vi "Calculate Center.vi"(8 "Type of Assembly Tray":i32, 9 "Syringe Coordinates":dbl[](array[numeric]), 10 "Relative Coordinates":dbl[][](array[numeric]), 11 "Fiducial Measurements":dbl[][](array[numeric])) -> (3 "XYZTheta Centers":dbl[][](array[numeric]) format="%#.9g")   [LabVIEW 2020, in "Assembly Tray.lvclass"]
uses:
  Assembly Tray.lvclass
  <vilib>/Analysis/NI_AALPro.lvlib
  <vilib>/Analysis/coordinate.llb/2D Cartesian Coordinate Rotation (Scalar).vi
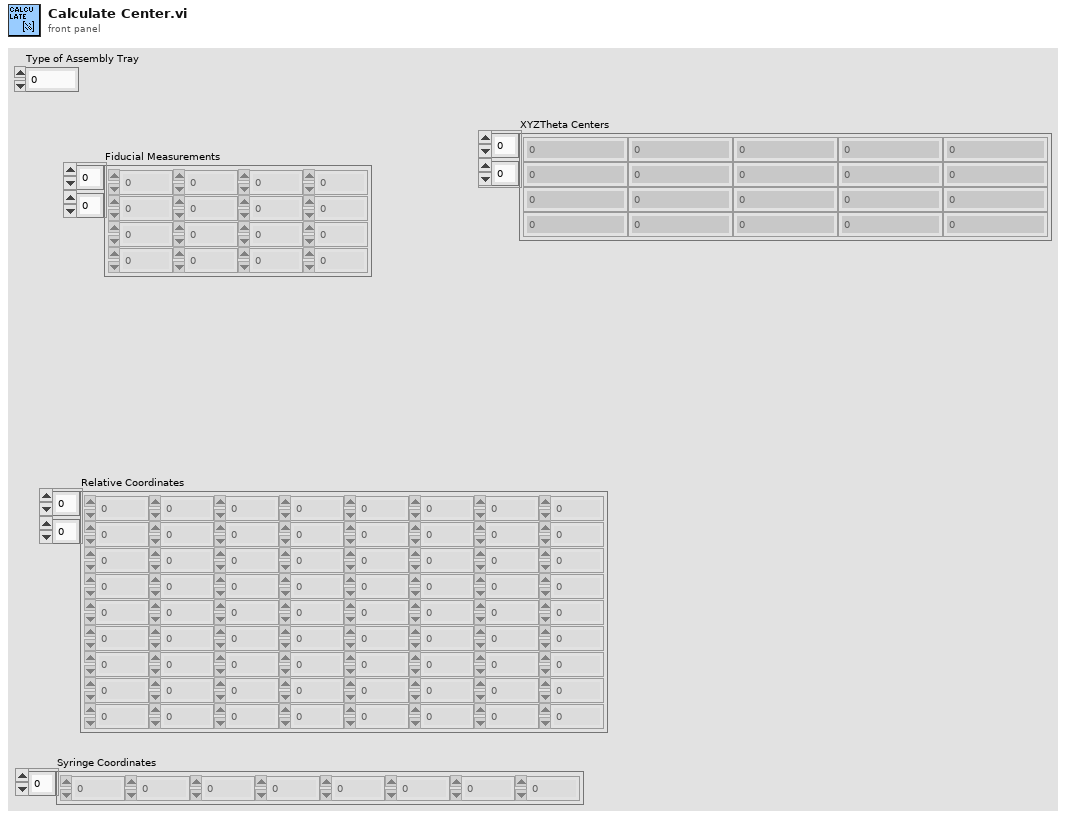
[diagram p1: front panel]
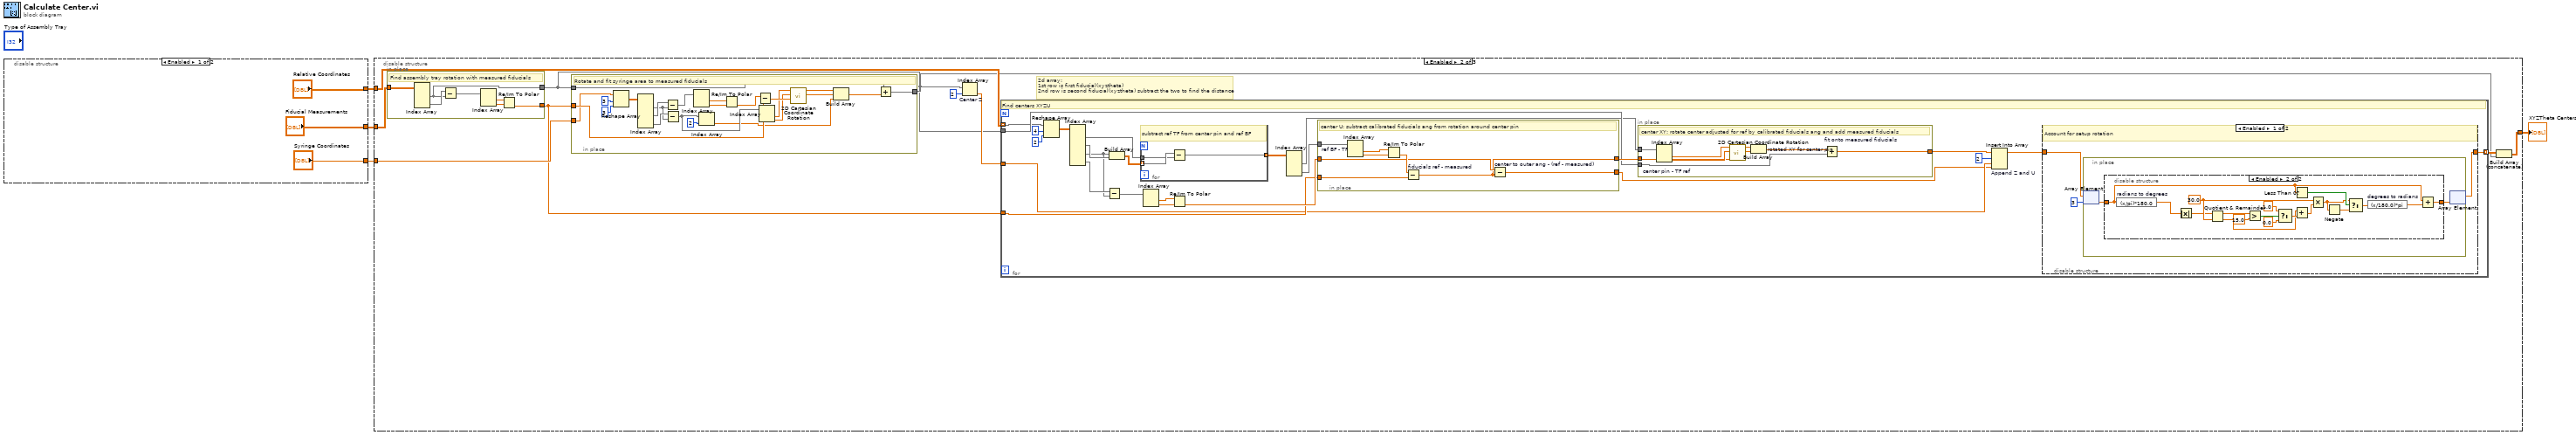
[diagram p0: block diagram]
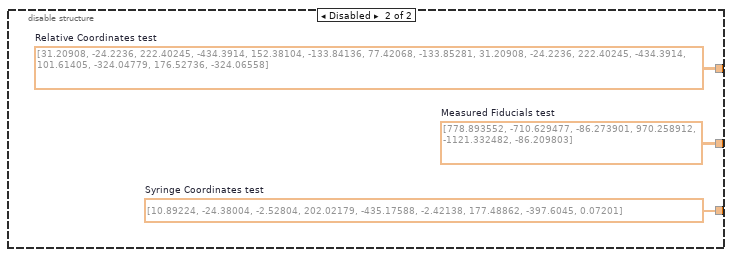
[diagram p2: hidden frame]
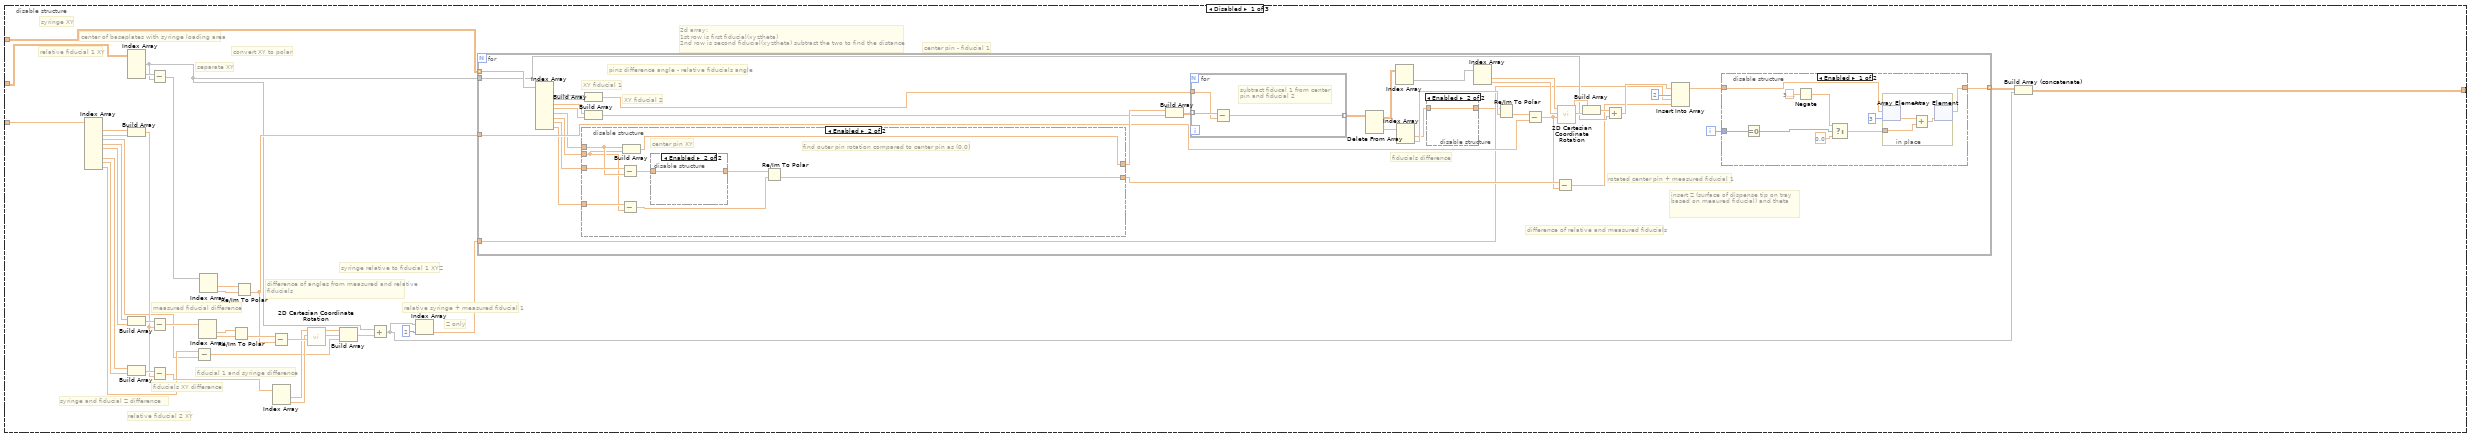
[diagram p3: hidden frame]
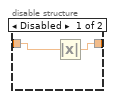
[diagram p4: hidden frame]
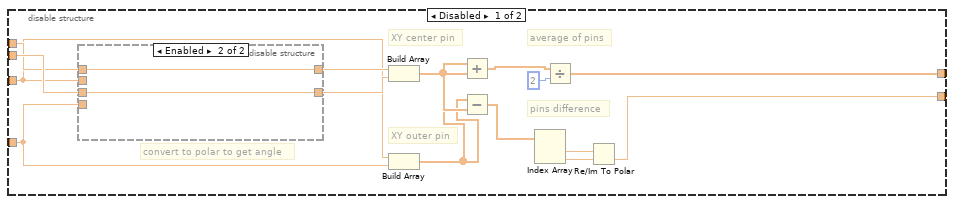
[diagram p5: hidden frame]
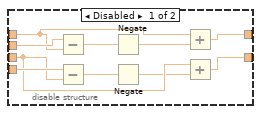
[diagram p6: hidden frame]
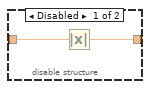
[diagram p7: hidden frame]
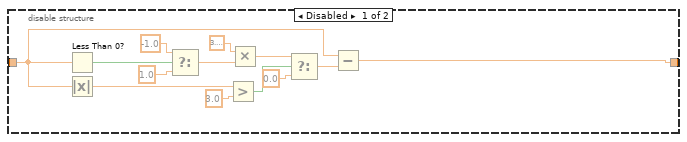
[diagram p9: hidden frame]
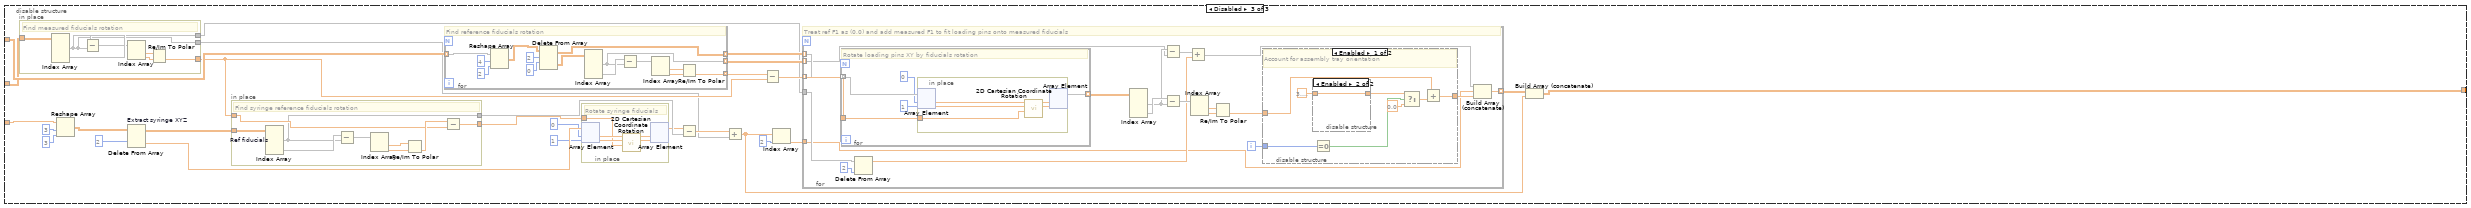
[diagram p11: hidden frame]
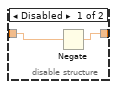
[diagram p12: hidden frame]
diagram:
  n1 = disable-structure shown="Enabled" {
    disable-tunnel: ["Syringe Coordinates" w8] -> w3
    disable-tunnel: ["Fiducial Measurements" w9] -> w2
    disable-tunnel: ["Relative Coordinates" w10] -> w1
    frame Enabled {
    }
    frame Disabled {
      w8 = dbl[] [10.89224, -24.38004, -2.52804, 202.02179, -435.17588, -2.42138, 177.48862, -397.6045, 0.07201]  # Syringe Coordinates test
      w9 = dbl[][] [[778.893552, -710.629477, -86.273901], [970.258912, -1121.332482, -86.209803]]  # Measured Fiducials test
      w10 = dbl[][] [[31.20908, -24.2236, 222.40245, -434.3914, 152.38104, -133.84136, 77.42068, -133.85281], [31.20908, -24.2236, 222.40245, -434.3914, 101.61405, -324.04779, 176.52736, -324.06558]]  # Relative Coordinates test
    }
  }
  n2 = disable-structure shown="Enabled" {
    disable-tunnel: w1 -> [w47 w152 w291]
    disable-tunnel: w2 -> [w44 w151 w290]
    disable-tunnel: w3 -> [w43 w150 w284]
    disable-tunnel: [w19 w147 w269] -> w4
    frame Disabled {
      # "center of baseplates with syringe loading area"
      # "relative fiducial 2 XY"
      # "relative fiducial 1 XY"
      # "syringe XY"
      # "center pin - fiducial 1"
      # "Z only"
      # "relative syringe + measured fiducial 1"
      # "syringe relative to fiducial 1 XYZ"
      # "difference of angles from measured and relative fiducials"
      # "separate XY"
      # "convert XY to polar"
      # "measured fiducial difference"
      # "fiducial 1 and syringe difference"
      # "syringe and fiducial Z difference"
      # "fiducials XY difference"
      # "2d array:\n1st row is first fiducial(xyztheta)\n2nd row is second fiducial(xyztheta) subtract the two to find the distance"
      n3 = Index Array(array=w43) -> (element #1=w42:dbl, element #2=w41:dbl, element #3=w23:dbl, element #4=w39:dbl, element #5=w38:dbl, element #7=w26:dbl, element #8=w25:dbl, element #9=w24:dbl)  [unwired: 9 in, 1 out]
      n4 = Index Array(array=w44) -> (element #1=w11:dbl[], element #2=w13:dbl[])  [unwired: 4 in]
      n5 = Build Array(w42, w41) -> (w30:dbl[])
      n6 = Build Array(w39, w38) -> (w40:dbl[])
      n7 = Build Array(w26, w25) -> (w31:dbl[])
      n8 = Subtract(x=w13, y=w11) -> (x-y=w18:dbl[])
      n9 = Subtract(x=w40, y=w30) -> (x-y=w37:dbl[])
      n10 = Subtract(x=w31, y=w30) -> (x-y=w29:dbl[])
      n11 = Subtract(x=w24, y=w23) -> (x-y=w15:dbl)
      n12 = Index Array(array=w37) -> (element #1=w36:dbl, element #2=w35:dbl)  [unwired: 2 in]
      n13 = Index Array(array=w18) -> (element #1=w45:dbl, element #2=w46:dbl)  [unwired: 2 in]
      n14 = Re/Im To Polar(2:w35, 3:w36) -> (0:w34:dbl)  [unwired: 1 out]
      n15 = Re/Im To Polar(2:w46, 3:w45) -> (0:w33:dbl)  [unwired: 1 out]
      n16 = Subtract(x=w34, y=w33) -> (x-y=w32:dbl)
      n17 = Index Array(array=w29) -> (element #1=w28:dbl, element #2=w27:dbl)  [unwired: 2 in]
      n18 = call-poly <vilib>:"2D Cartesian Coordinate Rotation.vi"("theta"=w32, "y"=w27, "x"=w28) -> ("y out"=w21:dbl, "x out"=w22:dbl)  [unwired: 6 in, 1 out]
      n19 = Build Array(w22, w21, w15) -> (w12:dbl[])
      n20 = Add(x=w11, y=w12) -> (x+y=w14:dbl[])
      n21 = Index Array(array=w14, index=2) -> (element=w16:dbl)
      n22 = for {
        tunnel: w47 -> [w64] mode=indexing
        tunnel: [w55] -> w20 mode=indexing
        tunnel: w11 -> [w63]
        tunnel: w33 -> [w62]
        tunnel: w16 -> [w61]
        i -> [w54]
        # "insert Z (surface of dispense tip on tray based on meaured fiducial) and theta"
        # "pins difference angle - relative fiducials angle"
        # "rotated center pin + measured fiducial 1"
        # "difference of relative and measured fiducials"
        # "fiducials difference"
        # "XY fiducial 2"
        # "XY fiducial 1"
        n23 = Index Array(array=w64) -> (element #1=w84:dbl, element #2=w83:dbl, element #3=w53:dbl, element #4=w52:dbl, element #5=w59:dbl, element #6=w60:dbl, element #7=w58:dbl, element #8=w57:dbl)  [unwired: 8 in]
        n24 = disable-structure shown="Enabled" {
          disable-tunnel: [w100 w115] -> w68
          disable-tunnel: [w94 w119] -> w66
          disable-tunnel: w60 -> [w91 w116]
          disable-tunnel: w59 -> [w90 w117]
          disable-tunnel: w58 -> [w89 w120]
          disable-tunnel: w57 -> [w88 w118]
          frame Disabled {
            # "convert to polar to get angle"
            # "pins difference"
            # "average of pins"
            # "XY outer pin"
            # "XY center pin"
            n25 = disable-structure shown="Enabled" {
              disable-tunnel: w88 -> [w112 _]
              disable-tunnel: w89 -> [w111 _]
              disable-tunnel: w91 -> [w108 w114]
              disable-tunnel: w90 -> [w105 w113]
              disable-tunnel: [w104 w114] -> w92
              disable-tunnel: [w103 w113] -> w93
              frame Disabled {
                n26 = Subtract(x=w111, y=w105) -> (x-y=w109:dbl)
                n27 = Subtract(x=w112, y=w108) -> (x-y=w110:dbl)
                n28 = Negate(x=w109) -> (-x=w106:dbl)
                n29 = Negate(x=w110) -> (-x=w107:dbl)
                n30 = Add(x=w105, y=w106) -> (x+y=w103:dbl)
                n31 = Add(x=w108, y=w107) -> (x+y=w104:dbl)
              }
              frame Enabled {
              }
            }
            n32 = Build Array(w93, w92) -> (w99:dbl[])
            n33 = Build Array(w89, w88) -> (w98:dbl[])
            n34 = Add(x=w98, y=w99) -> (x+y=w101:dbl[])
            n35 = Subtract(x=w98, y=w99) -> (x-y=w97:dbl[])
            n36 = Index Array(array=w97) -> (element #1=w96:dbl, element #2=w95:dbl)  [unwired: 2 in]
            n37 = Divide(x=w101, y=2) -> (x/y=w100:dbl[])
            n38 = Re/Im To Polar(2:w95, 3:w96) -> (0:w94:dbl)  [unwired: 1 out]
          }
          frame Enabled {
            # "find outer pin rotation compared to center pin as (0,0)"
            # "center pin XY"
            n39 = Subtract(x=w120, y=w117) -> (x-y=w122:dbl)
            n40 = Subtract(x=w118, y=w116) -> (x-y=w123:dbl)
            n41 = Build Array(w117, w116) -> (w115:dbl[])
            n42 = disable-structure shown="Enabled" {
              disable-tunnel: w122 -> [w125 w126]
              disable-tunnel: [w124 w126] -> w121
              frame Disabled {
                n43 = Absolute Value(x=w125) -> (abs(x)=w124:dbl)
              }
              frame Enabled {
              }
            }
            n44 = Re/Im To Polar(2:w123, 3:w121) -> (0:w119:dbl)  [unwired: 1 out]
          }
        }
        n45 = Build Array(w84, w83) -> (w81:dbl[])
        n46 = Build Array(w53, w52) -> (w51:dbl[])
        n47 = Build Array(w68, w51) -> (w82:dbl[][])
        n48 = for {
          tunnel: w82 -> [w142] mode=indexing
          tunnel: w81 -> [w141]
          tunnel: [w140] -> w80 mode=indexing
          # "subtract fiducal 1 from center pin and fiducial 2"
          n49 = Subtract(x=w142, y=w141) -> (x-y=w140:dbl[])
        }
        n50 = Delete From Array(array=w80) -> (deleted portion=w79:dbl[], array with subset deleted=w77:dbl[][])  [unwired: 3 in]
        n51 = Index Array(array=w77) -> (element=w76:dbl[])  [unwired: 2 in]
        n52 = Index Array(array=w79) -> (element #1=w50:dbl, element #2=w78:dbl)  [unwired: 2 in]
        n53 = disable-structure shown="Enabled" {
          disable-tunnel: w50 -> [w86 w87]
          disable-tunnel: [w85 w87] -> w49
          frame Disabled {
            n54 = Absolute Value(x=w86) -> (abs(x)=w85:dbl)
          }
          frame Enabled {
          }
        }
        n55 = Index Array(array=w76) -> (element #1=w75:dbl, element #2=w74:dbl)  [unwired: 2 in]
        n56 = Re/Im To Polar(2:w78, 3:w49) -> (0:w67:dbl)  [unwired: 1 out]
        n57 = Subtract(x=w67, y=w62) -> (x-y=w65:dbl)
        n58 = Subtract(x=w66, y=w65) -> (x-y=w48:dbl)
        n59 = call-poly <vilib>:"2D Cartesian Coordinate Rotation.vi"("theta"=w65, "y"=w74, "x"=w75) -> ("y out"=w71:dbl, "x out"=w72:dbl)  [unwired: 6 in, 1 out]
        n60 = Build Array(w72, w71) -> (w73:dbl[])
        n61 = Add(x=w73, y=w63) -> (x+y=w70:dbl[])
        n62 = Insert Into Array(array=w70, index=2, new element #1=w61, new element #2=w48) -> (w56:dbl[])
        n63 = disable-structure shown="Enabled" {
          disable-tunnel: w56 -> [w135 w139]
          disable-tunnel: [w134 w139] -> w55
          disable-tunnel: w54 -> [w132 _]
          frame Enabled {
            n64 = Equal To 0?(x=w132) -> (x = 0?=w130:bool)
            n65 = Negate(x=3.141592653589793) -> (-x=w127:dbl)
            n66 = Select(t=w127, s=w130, f=0.0) -> (s? t:f=w129:dbl)
            n67 = in-place {
              in-place-border: w129 -> [w136]
              n68 = in-place-array #1(w135, 3) -> (w138:dbl)
              n69 = Add(x=w138, y=w136) -> (x+y=w137:dbl)
              n70 = in-place-array #1(w137) -> (w134:dbl[])  [unwired: 1 out]
            }
          }
          frame Disabled {
          }
        }
      }
      n71 = Build Array (concatenate)(w20, w14) -> (w19:dbl[][])
    }
    frame Enabled {
      # "2d array:\n1st row is first fiducial(xyztheta)\n2nd row is second fiducial(xyztheta) subtract the two to find the distance"
      n72 = in-place {
        in-place-border: w151 -> [w239]
        in-place-border: [w238] -> w149
        in-place-border: [w235] -> w143
        # "Find assembly tray rotation with measured fiducials"
        n73 = Index Array(array=w239) -> (element #1=w235:dbl[], element #2=w236:dbl[])  [unwired: 4 in]
        n74 = Subtract(x=w236, y=w235) -> (x-y=w237:dbl[])
        n75 = Index Array(array=w237) -> (element #1=w240:dbl, element #2=w241:dbl)  [unwired: 2 in]
        n76 = Re/Im To Polar(2:w241, 3:w240) -> (0:w238:dbl)  [unwired: 1 out]
      }
      n77 = in-place {
        in-place-border: w150 -> [w252]
        in-place-border: w149 -> [w261]
        in-place-border: [w255] -> w144
        in-place-border: w143 -> [w253]
        # "Rotate and fit syringe area to measured fiducials"
        n78 = Reshape Array(w252, 3 ("dimension size"), 3 ("dimension size")) -> (w249:dbl[][])
        n79 = Index Array(array=w249) -> (element #1=w246:dbl[], element #2=w248:dbl[], element #3=w247:dbl[])  [unwired: 6 in]
        n80 = Subtract(x=w248, y=w246) -> (x-y=w245:dbl[])
        n81 = Subtract(x=w247, y=w246) -> (x-y=w244:dbl[])
        n82 = Index Array(array=w245) -> (element #1=w264:dbl, element #2=w263:dbl)  [unwired: 2 in]
        n83 = Index Array(array=w244, index=2) -> (element=w242:dbl)
        n84 = Re/Im To Polar(2:w263, 3:w264) -> (0:w262:dbl)  [unwired: 1 out]
        n85 = Subtract(x=w262, y=w261) -> (x-y=w260:dbl)
        n86 = Index Array(array=w244) -> (element #1=w259:dbl, element #2=w258:dbl)  [unwired: 2 in]
        n87 = call-poly <vilib>:"2D Cartesian Coordinate Rotation.vi"("theta"=w260, "y"=w258, "x"=w259) -> ("y out"=w256:dbl, "x out"=w257:dbl)  [unwired: 6 in, 1 out]
        n88 = Build Array(w257, w256, w242) -> (w254:dbl[])
        n89 = Add(x=w253, y=w254) -> (x+y=w255:dbl[])
      }
      n90 = Index Array "Center Z"(array=w144, index=2) -> (element=w145:dbl)
      n91 = for {
        tunnel: w152 -> [w166] mode=indexing
        tunnel: [w168] -> w148 mode=indexing
        tunnel: w143 -> [w172]
        tunnel: w149 -> [w171]
        tunnel: w145 -> [w170]
        # "Find centers XYZU"
        n92 = Reshape Array(w166, 4 ("dimension size"), 2 ("dimension size")) -> (w163:dbl[][])
        n93 = Index Array(array=w163) -> (element #1=w158:dbl[], element #2=w157:dbl[], element #3=w156:dbl[], element #4=w162:dbl[])  [unwired: 8 in]
        n94 = Subtract(x=w162, y=w156) -> (x-y=w161:dbl[])
        n95 = Build Array(w156, w157) -> (w177:dbl[][])
        n96 = for {
          tunnel: w177 -> [w234] mode=indexing
          tunnel: w158 -> [w233]
          tunnel: [w232] -> w155 mode=indexing
          # "subtract ref TF from center pin and ref BF"
          n97 = Subtract(x=w234, y=w233) -> (x-y=w232:dbl[])
        }
        n98 = Index Array(array=w161) -> (element #1=w160:dbl, element #2=w159:dbl)  [unwired: 2 in]
        n99 = Re/Im To Polar(2:w159, 3:w160) -> (0:w174:dbl)  [unwired: 1 out]
        n100 = Index Array(array=w155) -> (element #1=w154:dbl[], element #2=w153:dbl[])  [unwired: 4 in]
        n101 = in-place {
          in-place-border: w174 -> [w183]
          in-place-border: [w182] -> w173
          in-place-border: w171 -> [w181]
          in-place-border: [w179] -> w167
          in-place-border: w153 -> [w178]
          # "center U: subtract calibrated fiducials ang from rotation around center pin"
          n102 = Index Array "ref BF - TF"(array=w178) -> (element #1=w180:dbl, element #2=w185:dbl)  [unwired: 2 in]
          n103 = Re/Im To Polar(2:w185, 3:w180) -> (0:w184:dbl)  [unwired: 1 out]
          n104 = Subtract "fiducials ref - measured"(x=w184, y=w181) -> (x-y=w182:dbl)
          n105 = Subtract "center to outer ang - (ref - measured)"(x=w183, y=w182) -> (x-y=w179:dbl)
        }
        n106 = in-place {
          in-place-border: [w189] -> w176
          in-place-border: w173 -> [w188]
          in-place-border: w172 -> [w187]
          in-place-border: w154 -> [w186]
          # "center XY: rotate center adjusted for ref by calibrated fiducials ang and add measured fiducials"
          n107 = Index Array "center pin - TF ref"(array=w186) -> (element #1=w194:dbl, element #2=w193:dbl)  [unwired: 2 in]
          n108 = call-poly <vilib>:"2D Cartesian Coordinate Rotation.vi"("theta"=w188, "y"=w193, "x"=w194) -> ("y out"=w190:dbl, "x out"=w191:dbl)  [unwired: 6 in, 1 out]
          n109 = Build Array "rotated XY for center pin"(w191, w190) -> (w192:dbl[])
          n110 = Add "fit onto measured fiducials"(x=w192, y=w187) -> (x+y=w189:dbl[])
        }
        n111 = Insert Into Array "Append Z and U"(array=w176, index=2, new element #1=w170, new element #2=w167) -> (w169:dbl[])
        n112 = disable-structure shown="Enabled" {
          disable-tunnel: w169 -> [w196 w231]
          disable-tunnel: [w195 w231] -> w168
          frame Enabled {
            # "Account for setup rotation"
            n113 = in-place {
              n114 = in-place-array #2(w196, 3) -> (w199:dbl)
              n115 = disable-structure shown="Enabled" {
                disable-tunnel: w199 -> [w206 w216]
                disable-tunnel: [w205 w215] -> w198
                frame Disabled {
                  n116 = Less Than 0?(x=w206) -> (x < 0?=w212:bool)
                  n117 = Absolute Value(x=w206) -> (abs(x)=w209:dbl)
                  n118 = Select(t=-1.0, s=w212, f=1.0) -> (s? t:f=w201:dbl)
                  n119 = Greater?(x=w209, y=3.0) -> (0:w207:bool)
                  n120 = Multiply(x=3.141592653589793, y=w201) -> (x*y=w200:dbl)
                  n121 = Select(t=w200, s=w207, f=0.0) -> (s? t:f=w203:dbl)
                  n122 = Subtract(x=w206, y=w203) -> (x-y=w205:dbl)
                }
                frame Enabled {
                  w223 = 30.0 ("y")
                  n123 = expression code="(x/pi)*180.0" "radians to degrees"(w216) -> (w214:dbl)
                  n124 = Absolute Value(x=w214) -> (abs(x)=w213:dbl)
                  n125 = Quotient & Remainder(x=w213, y=w223) -> (x-y*floor(x/y)=w230:dbl, floor(x/y)=w224:dbl)
                  n126 = Greater?(x=w230, y=15.0) -> (0:w228:bool)
                  n127 = Select(t=1.0, s=w228, f=0.0) -> (s? t:f=w225:dbl)
                  n128 = Less Than 0?(x=w216) -> (x < 0?=w221:bool)
                  n129 = Add(x=w224, y=w225) -> (x+y=w222:dbl)
                  n130 = Multiply(x=w223, y=w222) -> (x*y=w220:dbl)
                  n131 = Negate(x=w220) -> (-x=w219:dbl)
                  n132 = Select(t=w220, s=w221, f=w219) -> (s? t:f=w218:dbl)
                  n133 = expression code="(x/180.0)*pi" "degrees to radians"(w218) -> (w217:dbl)
                  n134 = Add(x=w216, y=w217) -> (x+y=w215:dbl)
                }
              }
              n135 = in-place-array #2(w198) -> (w195:dbl[])  [unwired: 1 out]
            }
          }
          frame Disabled {
          }
        }
      }
      n136 = Build Array (concatenate)(w148, w144) -> (w147:dbl[][])
    }
    frame Disabled {
      n137 = in-place {
        in-place-border: w290 -> [w306]
        in-place-border: [w308] -> w281
        in-place-border: [w307] -> w285
        in-place-border: [w307] -> w271
        # "Find measured fiducials rotation"
        n138 = Index Array(array=w306) -> (element #1=w307:dbl[], element #2=w312:dbl[])  [unwired: 4 in]
        n139 = Subtract(x=w312, y=w307) -> (x-y=w311:dbl[])
        n140 = Index Array(array=w311) -> (element #1=w310:dbl, element #2=w309:dbl)  [unwired: 2 in]
        n141 = Re/Im To Polar(2:w309, 3:w310) -> (0:w308:dbl)  [unwired: 1 out]
      }
      n142 = Reshape Array(w284, 3 ("dimension size"), 3 ("dimension size")) -> (w280:dbl[][])
      n143 = Delete From Array "Extract syringe XYZ"(array=w280, index (row)=2) -> (deleted portion=w277:dbl[], array with subset deleted=w278:dbl[][])  [unwired: 2 in]
      n144 = in-place {
        in-place-border: w281 -> [w300]
        in-place-border: w278 -> [w299]
        in-place-border: [w298] -> w274
        in-place-border: [w297] -> w273
        # "Find syringe reference fiducials rotation"
        n145 = Index Array "Ref fiducials"(array=w299) -> (element #1=w297:dbl[], element #2=w305:dbl[])  [unwired: 4 in]
        n146 = Subtract(x=w305, y=w297) -> (x-y=w304:dbl[])
        n147 = Index Array(array=w304) -> (element #1=w303:dbl, element #2=w302:dbl)  [unwired: 2 in]
        n148 = Re/Im To Polar(2:w302, 3:w303) -> (0:w301:dbl)  [unwired: 1 out]
        n149 = Subtract(x=w301, y=w300) -> (x-y=w298:dbl)
      }
      n150 = for {
        tunnel: w291 -> [w367] mode=indexing
        tunnel: [w360] -> w289 mode=indexing
        tunnel: [w359] -> w286 mode=indexing
        tunnel: [w355] -> w287 mode=indexing
        # "Find reference fiducials rotation"
        n151 = Reshape Array(w367, 4 ("dimension size"), 2 ("dimension size")) -> (w358:dbl[][])
        n152 = Delete From Array(array=w358, length=2, index (row)=0) -> (deleted portion=w354:dbl[][], array with subset deleted=w355:dbl[][])  [unwired: 1 in]
        n153 = Index Array(array=w354) -> (element #1=w359:dbl[], element #2=w364:dbl[])  [unwired: 4 in]
        n154 = Subtract(x=w364, y=w359) -> (x-y=w363:dbl[])
        n155 = Index Array(array=w363) -> (element #1=w362:dbl, element #2=w361:dbl)  [unwired: 2 in]
        n156 = Re/Im To Polar(2:w361, 3:w362) -> (0:w360:dbl)  [unwired: 1 out]
      }
      n157 = in-place {
        in-place-border: w274 -> [w294]
        # "Rotate syringe fiducials"
        n158 = in-place-array #3(w277, 0, 1) -> (w296:dbl, w295:dbl)
        n159 = call-poly <vilib>:"2D Cartesian Coordinate Rotation.vi"("theta"=w294, "y"=w295, "x"=w296) -> ("y out"=w292:dbl, "x out"=w293:dbl)  [unwired: 6 in, 1 out]
        n160 = in-place-array #3(w293, w292) -> (w270:dbl[])  [unwired: 2 out]
      }
      n161 = Subtract(x=w270, y=w273) -> (x-y=w272:dbl[])
      n162 = Add(x=w272, y=w271) -> (x+y=w267:dbl[])
      n163 = Subtract(x=w289, y=w281) -> (x-y=w288:dbl[])
      n164 = Index Array(array=w267, index=2) -> (element=w265:dbl)
      n165 = for {
        tunnel: w288 -> [w331] mode=indexing
        tunnel: w287 -> [w330] mode=indexing
        tunnel: [w324] -> w268 mode=indexing
        tunnel: w286 -> [w317] mode=indexing
        tunnel: w285 -> [w316]
        tunnel: w265 -> [w313]
        i -> [w323]
        # "Treat ref F1 as (0,0) and add measured F1 to fit loading pins onto measured fiducials"
        n166 = for {
          tunnel: w331 -> [w348]
          tunnel: w330 -> [w347] mode=indexing
          tunnel: [w344] -> w329 mode=indexing
          # "Rotate loading pins XY by fiducials rotation"
          n167 = in-place {
            in-place-border: w348 -> [w353]
            n168 = in-place-array #4(w347, 0, 1) -> (w352:dbl, w351:dbl)
            n169 = call-poly <vilib>:"2D Cartesian Coordinate Rotation.vi"("theta"=w353, "y"=w351, "x"=w352) -> ("y out"=w349:dbl, "x out"=w350:dbl)  [unwired: 6 in, 1 out]
            n170 = in-place-array #4(w350, w349) -> (w344:dbl[])  [unwired: 2 out]
          }
        }
        n171 = Delete From Array(array=w316, index=2) -> (array with subset deleted=w314:dbl[])  [unwired: 1 in, 1 out]
        n172 = Index Array(array=w329) -> (element #1=w318:dbl[], element #2=w328:dbl[])  [unwired: 4 in]
        n173 = Subtract(x=w318, y=w317) -> (x-y=w320:dbl[])
        n174 = Subtract(x=w328, y=w318) -> (x-y=w327:dbl[])
        n175 = Add(x=w320, y=w314) -> (x+y=w319:dbl[])
        n176 = Index Array(array=w327) -> (element #1=w326:dbl, element #2=w325:dbl)  [unwired: 2 in]
        n177 = Re/Im To Polar(2:w325, 3:w326) -> (0:w322:dbl)  [unwired: 1 out]
        n178 = disable-structure shown="Enabled" {
          disable-tunnel: w323 -> [w337 _]
          disable-tunnel: w322 -> [w336 w343]
          disable-tunnel: [w334 w343] -> w321
          frame Enabled {
            # "Account for assembly tray orientation"
            n179 = disable-structure shown="Enabled" {
              disable-tunnel: 3.141592653589793 -> [w341 w342]
              disable-tunnel: [w340 w342] -> w332
              frame Disabled {
                n180 = Negate(x=w341) -> (-x=w340:dbl)
              }
              frame Enabled {
              }
            }
            n181 = Equal To 0?(x=w337) -> (x = 0?=w339:bool)
            n182 = Select(t=w332, s=w339, f=0.0) -> (s? t:f=w335:dbl)
            n183 = Add(x=w336, y=w335) -> (x+y=w334:dbl)
          }
          frame Disabled {
          }
        }
        n184 = Build Array (concatenate)(w319, w313, w321) -> (w324:dbl[])
      }
      n185 = Build Array (concatenate)(w268, w267) -> (w269:dbl[][])
    }
  }
  "XYZTheta Centers" <- w4
